vi "Textures.vi"() -> ()   [LabVIEW 2020]
panel:
  in  "Tex 1 DVR":refnum<data-value>
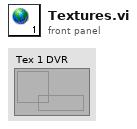
[diagram p1: front panel]
diagram:
